vi "Prepare_dataST.vi"(1 "Active Sensors":bool[](array[boolean]), 2 "ranges":bool[](array[boolean]), 3 "Controls[]":refnum<vi>[](array[refnum]), 4 "Flag_215":bool, 5 "error in":errorcluster, 7 "chkeach_ch":bool, 9 "chk2scan":bool) -> (12 "Meas_rang":i32[](array[numeric]), 13 "Refdata_struct":refnum<k24>[](array[refnum]), 15 "Meas_monitor_struct":refnum<k24>[](array[refnum]), 16 "Data_struct":refnum<k24>[](array[refnum]), 17 "Ref_monitordata_struct":refnum<k24>[](array[refnum]), 18 "Mergedata_struct":refnum<k24>[](array[refnum]), 19 "error out":errorcluster)   [LabVIEW 2017]
doc: "prepare data struct & hold instrument condition"
uses:
  D:/test/PDLSTS/LV_PDL LvVer17.0/LV_PDL_x86/DLL/STSProcess.dll
  DLL/STSProcess.dll
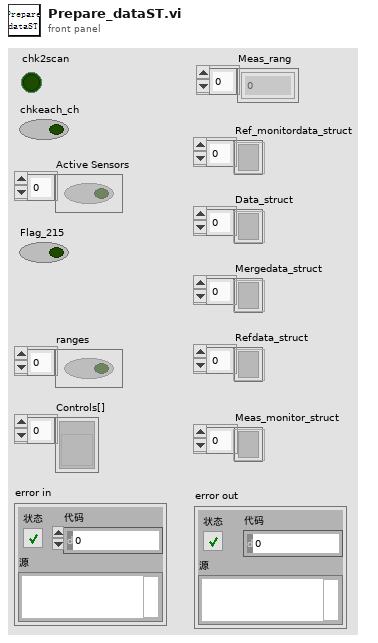
[diagram p1: front panel]
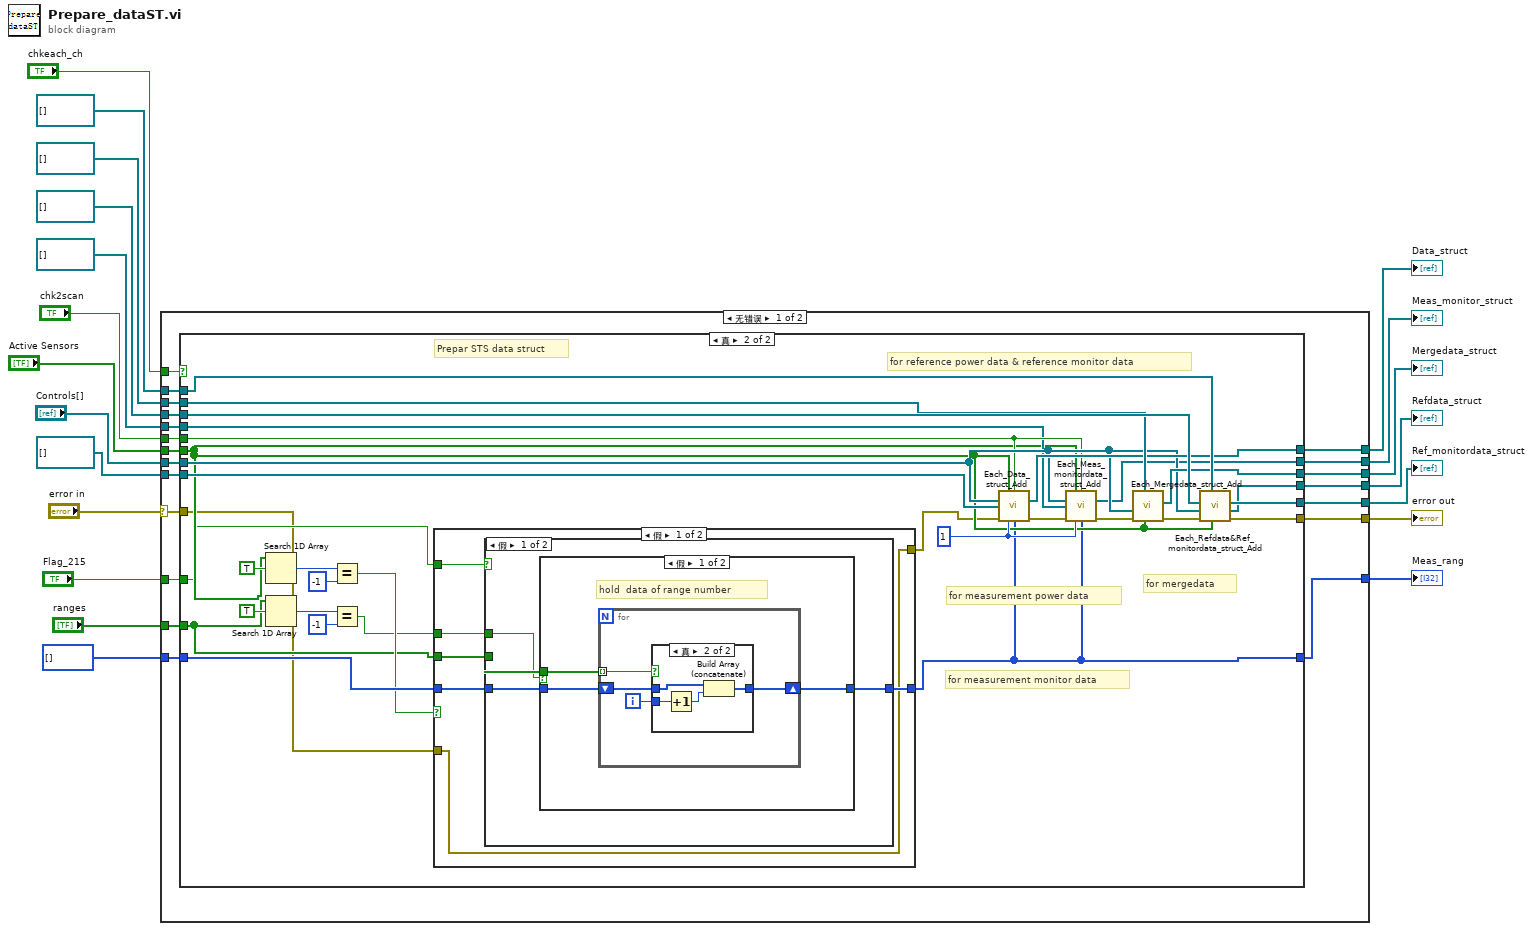
[diagram p0: block diagram]
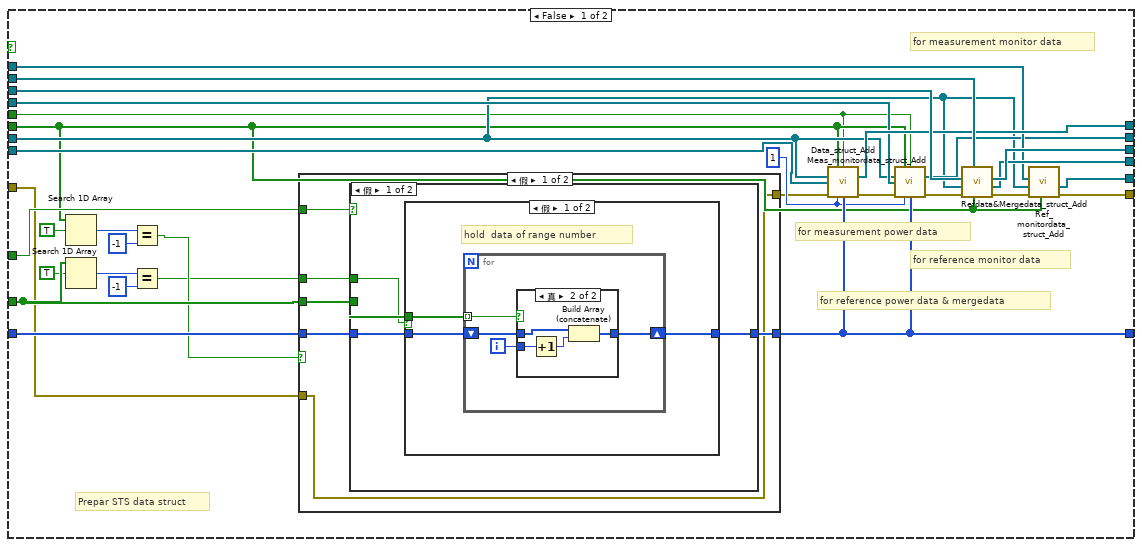
[diagram p2: hidden frame]
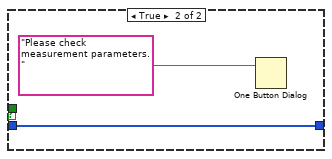
[diagram p4: hidden frame]
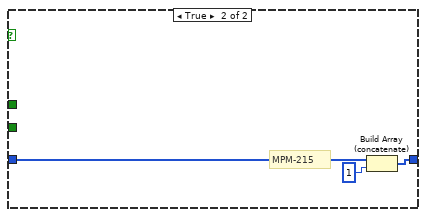
[diagram p5: hidden frame]
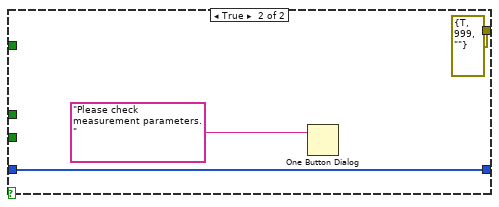
[diagram p6: hidden frame]
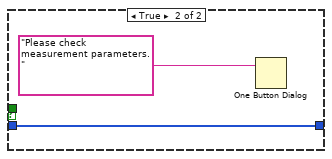
[diagram p8: hidden frame]
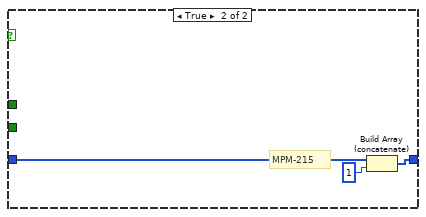
[diagram p9: hidden frame]
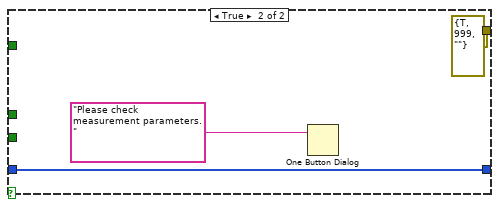
[diagram p10: hidden frame]
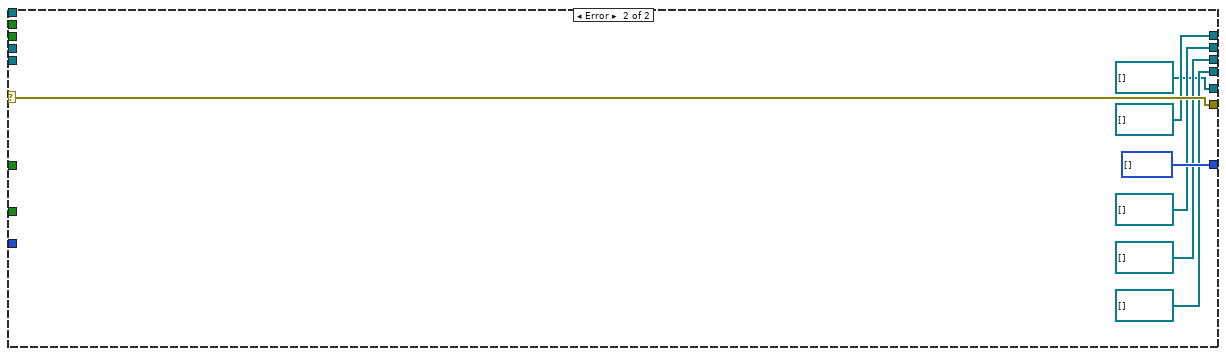
[diagram p11: hidden frame]
diagram:
  n1 = case shown="无错误" "error in" {
    selector: "error in" -> [w22 w171]
    tunnel: "ranges" -> [w40 _]
    tunnel: "Flag_215" -> [w39 _]
    tunnel: "Controls[]" -> [w38 _]
    tunnel: "Active Sensors" -> [w37 _]
    tunnel: "chkeach_ch" -> [w36 _]
    tunnel: refnum<k24>[] [] ("Data_struct") -> [w35 _]
    tunnel: refnum<k24>[] [] ("Ref_monitordata_struct") -> [w34 _]
    tunnel: refnum<k24>[] [] ("Mergedata_struct") -> [w33 _]
    tunnel: refnum<k24>[] [] ("Meas_monitor_struct") -> [w32 _]
    tunnel: refnum<k24>[] [] ("Refdata_struct") -> [w31 _]
    tunnel: [w30 refnum<k24>[] [] ("Mergedata_struct")] -> w10
    tunnel: [w29 refnum<k24>[] [] ("Data_struct")] -> w9
    tunnel: [w28 refnum<k24>[] [] ("Meas_monitor_struct")] -> w8
    tunnel: [w27 refnum<k24>[] [] ("Refdata_struct")] -> w7
    tunnel: [w26 refnum<k24>[] [] ("Ref_monitordata_struct")] -> w6
    tunnel: i32[] [] ("Meas_rang") -> [w25 _]
    tunnel: [w24 i32[] [] ("Meas_rang")] -> w4
    tunnel: [w23 w171] -> w2
    tunnel: "chk2scan" -> [w21 _]
    frame No Error {
      n2 = case shown="真" w36 {
        tunnel: w37 -> [w53 w110]
        tunnel: w38 -> [w54 w122]
        tunnel: w35 -> [w72 w127]
        tunnel: w32 -> [w58 w119]
        tunnel: w31 -> [w71 w131]
        tunnel: w33 -> [w70 w129]
        tunnel: w34 -> [w62 w133]
        tunnel: w25 -> [w69 w117]
        tunnel: w39 -> [w68 w106]
        tunnel: w40 -> [w67 w107]
        tunnel: [w66 w128] -> w30
        tunnel: [w65 w126] -> w29
        tunnel: [w59 w118] -> w28
        tunnel: [w64 w130] -> w27
        tunnel: [w63 w132] -> w26
        tunnel: [w55 w105] -> w24
        tunnel: [w60 w124] -> w23
        tunnel: w22 -> [w44 w104]
        tunnel: w21 -> [w52 w121]
        frame False {
          w51 = 1 ("sweep_count")
          # "for measurement monitor data"
          # "for measurement power data"
          # "for reference power data & mergedata"
          # "for reference monitor data"
          # "Prepar STS data struct"
          n3 = Search 1D Array(1D array=w53, element=TRUE ("元素")) -> (index of element=w49:i32)  [unwired: 1 in]
          n4 = Search 1D Array(1D array=w67, element=TRUE ("元素")) -> (index of element=w50:i32)  [unwired: 1 in]
          n5 = Equal?(x=w49, y=-1) -> (x = y?=w42:bool)
          n6 = Equal?(x=w50, y=-1) -> (x = y?=w41:bool)
          n7 = case shown="假" w42 {
            tunnel: w69 -> [w78 w101]
            tunnel: w68 -> [w77 _]
            tunnel: w67 -> [w76 _]
            tunnel: [w75 w101] -> w55
            tunnel: w44 -> [w74 _]
            tunnel: [w74 errorcluster {"status"=TRUE, "code"=999, "source"=""} ("error IO")] -> w43
            tunnel: w41 -> [w73 _]
            frame False {
              n8 = case shown="假" w77 {
                tunnel: w78 -> [w82 w99]
                tunnel: [w81 w97] -> w75
                tunnel: w76 -> [w80 _]
                tunnel: w73 -> [w79 _]
                frame False {
                  n9 = case shown="假" w79 {
                    tunnel: w82 -> [w85 w95]
                    tunnel: [w84 w95] -> w81
                    tunnel: w80 -> [w83 _]
                    frame False {
                      # "hold  data of range number"
                      n10 = for {
                        tunnel: w83 -> [w89] mode=indexing
                        shift-right: [w86] -> w84
                        shift-left: w85 -> [w88]
                        i -> [w87]
                        n11 = case shown="真" w89 {
                          tunnel: w88 -> [w90 w94]
                          tunnel: w87 -> [_ w92]
                          tunnel: [w90 w91] -> w86
                          frame False {
                          }
                          frame True {
                            n12 = Increment(x=w92) -> (x+1=w93:i32)
                            n13 = Build Array (concatenate)(w94, w93) -> (w91:i32[])
                          }
                        }
                      }
                    }
                    frame True {
                      n14 = One Button Dialog(message="Please check measurement parameters." ("消息")) -> ()  [unwired: 1 in, 1 out]
                    }
                  }
                }
                frame True {
                  # "MPM-215"
                  n15 = Build Array (concatenate)(w99, 1) -> (w97:i32[])
                }
              }
            }
            frame True {
              n16 = One Button Dialog(message="Please check measurement parameters." ("消息")) -> ()  [unwired: 1 in, 1 out]
            }
          }
          n17 = call "Data_struct_Add.vi"("Active Sensors"=w53, "chk2scan"=w52, "Controls[]"=w54, "Data_struct输入"=w72, "错误输入（无错误）"=w43, "sweep_count"=w51, "Meas_rang"=w55) -> ("Data_struct输出"=w65:refnum<k24>[], "错误输出"=w57:errorcluster)  [unwired: 7 in]
          n18 = call "Meas_monitordata_struct_Add.vi"("Active Sensors"=w53, "chk2scan"=w52, "Controls[]"=w54, "Meas_monitordata_struct输入"=w58, "错误输入（无错误）"=w57, "sweep_count"=w51, "Meas_rang"=w55) -> ("Meas_monitordata_struct输出"=w59:refnum<k24>[], "错误输出"=w56:errorcluster)  [unwired: 7 in]
          n19 = call "Refdata&Mergedata_struct_Add.vi"("Active Sensors"=w53, "Mergedata_struct输入"=w70, "错误输入（无错误）"=w56, "Controls[]"=w54, "Refdata_struct输入"=w71) -> ("错误输出"=w61:errorcluster, "Refdata_struct输出"=w64:refnum<k24>[], "Mergedata_struct输出"=w66:refnum<k24>[])  [unwired: 4 in]
          n20 = call "Ref_monitordata_struct_Add.vi"("Active Sensors"=w53, "错误输入（无错误）"=w61, "Controls[]"=w54, "Ref_monitordata_struct"=w62) -> ("错误输出"=w60:errorcluster, "Ref_monitordata_struct"=w63:refnum<k24>[])  [unwired: 6 in]
        }
        frame True {
          w125 = 1 ("sweep_count")
          # "for reference power data & reference monitor data"
          # "for mergedata"
          # "for measurement monitor data"
          # "for measurement power data"
          # "Prepar STS data struct"
          n21 = Search 1D Array(1D array=w110, element=TRUE ("元素")) -> (index of element=w115:i32)  [unwired: 1 in]
          n22 = Search 1D Array(1D array=w107, element=TRUE ("元素")) -> (index of element=w116:i32)  [unwired: 1 in]
          n23 = Equal?(x=w115, y=-1) -> (x = y?=w109:bool)
          n24 = Equal?(x=w116, y=-1) -> (x = y?=w108:bool)
          n25 = case shown="假" w109 {
            tunnel: w117 -> [w140 w163]
            tunnel: w106 -> [w139 _]
            tunnel: w107 -> [w138 _]
            tunnel: [w137 w163] -> w105
            tunnel: w104 -> [w136 _]
            tunnel: [w136 errorcluster {"status"=TRUE, "code"=999, "source"=""} ("error IO")] -> w103
            tunnel: w108 -> [w135 _]
            frame False {
              n26 = case shown="假" w139 {
                tunnel: w140 -> [w144 w161]
                tunnel: [w143 w159] -> w137
                tunnel: w138 -> [w142 _]
                tunnel: w135 -> [w141 _]
                frame False {
                  n27 = case shown="假" w141 {
                    tunnel: w144 -> [w147 w157]
                    tunnel: [w146 w157] -> w143
                    tunnel: w142 -> [w145 _]
                    frame False {
                      # "hold  data of range number"
                      n28 = for {
                        tunnel: w145 -> [w151] mode=indexing
                        shift-right: [w148] -> w146
                        shift-left: w147 -> [w150]
                        i -> [w149]
                        n29 = case shown="真" w151 {
                          tunnel: w150 -> [w152 w156]
                          tunnel: w149 -> [_ w154]
                          tunnel: [w152 w153] -> w148
                          frame False {
                          }
                          frame True {
                            n30 = Increment(x=w154) -> (x+1=w155:i32)
                            n31 = Build Array (concatenate)(w156, w155) -> (w153:i32[])
                          }
                        }
                      }
                    }
                    frame True {
                      n32 = One Button Dialog(message="Please check measurement parameters." ("消息")) -> ()  [unwired: 1 in, 1 out]
                    }
                  }
                }
                frame True {
                  # "MPM-215"
                  n33 = Build Array (concatenate)(w161, 1) -> (w159:i32[])
                }
              }
            }
            frame True {
              n34 = One Button Dialog(message="Please check measurement parameters." ("消息")) -> ()  [unwired: 1 in, 1 out]
            }
          }
          n35 = call "Each_Data_struct_Add.vi"("Active Sensors"=w110, "chk2scan"=w121, "Controls[]"=w122, "Data_struct输入"=w127, "错误输入（无错误）"=w103, "sweep_count"=w125, "Meas_rang"=w105) -> ("Data_struct输出"=w126:refnum<k24>[], "错误输出"=w123:errorcluster)  [unwired: 7 in]
          n36 = call "Each_Meas_monitordata_struct_Add.vi"("Active Sensors"=w110, "chk2scan"=w121, "Controls[]"=w122, "Meas_monitordata_struct输入"=w119, "错误输入（无错误）"=w123, "sweep_count"=w125, "Meas_rang"=w105) -> ("Meas_monitordata_struct输出"=w118:refnum<k24>[], "错误输出"=w120:errorcluster)  [unwired: 7 in]
          n37 = call "Each_Mergedata_struct_Add.vi"("Active Sensors"=w110, "Mergedata_struct输入"=w129, "错误输入（无错误）"=w120, "Controls[]"=w122) -> ("错误输出"=w134:errorcluster, "Mergedata_struct输出"=w128:refnum<k24>[])  [unwired: 6 in]
          n38 = call "Each_Refdata&Ref_monitordata_struct_Add.vi"("Active Sensors"=w110, "Ref_monitordata_struct输入"=w133, "错误输入（无错误）"=w134, "Controls[]"=w122, "Refdata_struct输入"=w131) -> ("错误输出"=w124:errorcluster, "Refdata_struct输出"=w130:refnum<k24>[], "Ref_monitordata_struct输出"=w132:refnum<k24>[])  [unwired: 4 in]
        }
      }
    }
    frame Error {
    }
  }
  "Ref_monitordata_struct" <- w6
  "Mergedata_struct" <- w10
  "Refdata_struct" <- w7
  "Meas_monitor_struct" <- w8
  "Data_struct" <- w9
  "Meas_rang" <- w4
  "error out" <- w2
